vi "Set_Parameter_Instrument (Json).vi"(8 "error in (no error)":errorcluster caption="entrée d'erreur (pas d'erreur)", 10 "Parameter (Json)":string, 11 "Flash_SIN_FP en entrée":refnum<class "Flash_SIN_Test_FW.lvclass">) -> (0 "error out":errorcluster caption="sortie d'erreur", 3 "Flash_SIN_FP en sortie":refnum<class "Flash_SIN_Test_FW.lvclass">)   [LabVIEW 2020, in "Library Test.lvlib" / "Flash_SIN_Test_FW.lvclass"]
uses:
  Flash_SIN_Test_FW.lvclass
  C:/Users/ngarcin/OneDrive - Altyor/Standard TB/Class/Test/Test (Default)/Test (Default).lvclass
  C:/Users/ngarcin/OneDrive - Altyor/Standard TB/Class/Test/Flash_Commander/Flash_Commander.lvclass
  Flash_SIN_Test_FW.lvclass/Flash_SIN_Test_FW.ctl
  JSON API/JSON Value/Set from JSON string.vi
  Flash_Commander/Flash_Commander.lvclass
  JSON API/JSON Value/JSON Value.lvclass
  JSON API/Variant JSON/Variant JSON.lvlib
  JSON API/Get Polymorphic/JSON GetSet.lvlib
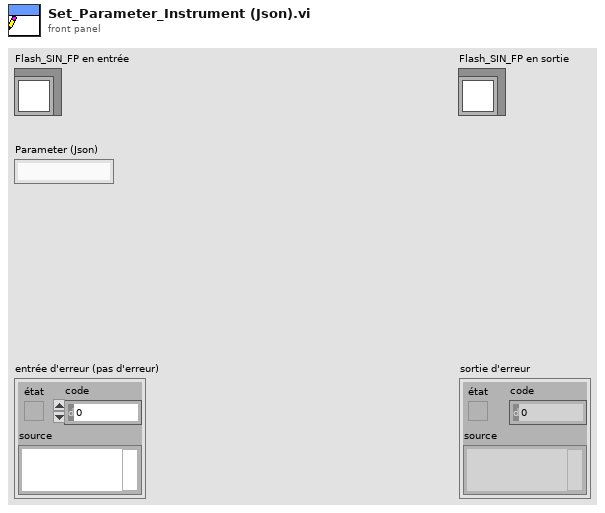
[diagram p1: front panel]
types:
  T1 = cluster{"Firmware path":path, "commander path":path, "Bat path":path}
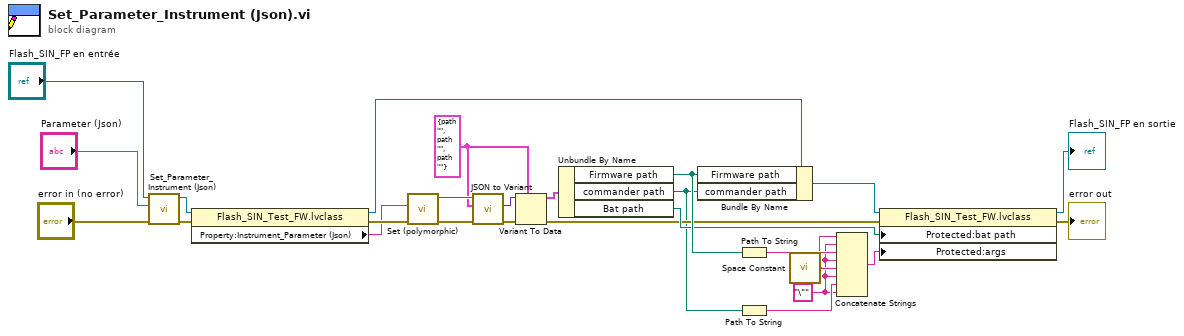
[diagram p0: block diagram]
diagram:
  w1 = "\""
  w13 = T1 {"Firmware path"=path "", "commander path"=path "", "Bat path"=path ""} ("Cluster des données privées de classe")
  n1 = call-parent "Set_Parameter_Instrument (Json).vi"("error in (no error)"="error in (no error)", "Parameter (Json)"="Parameter (Json)", "Test (Default) en entrée"="Flash_SIN_FP en entrée") -> ("error out"=w21:errorcluster, "Test (Default) en sortie"=w20:refnum<class "Flash_SIN_Test_FW.lvclass">)  [unwired: 7 in]
  n2 = property class="Flash_SIN_Test_FW.lvclass"(reference=w20, error in=w21) -> (reference out=w16:refnum<class "Flash_SIN_Test_FW.lvclass">, error out=w19:errorcluster, "Property:Instrument_Parameter (Json)"=w17:string)
  n3 = call-poly "Set (polymorphic).vi"("error in (no error)"=w19, "JSON stream"=w17) -> ("error out"=w24:errorcluster, "JSON Value out"=w26:refnum<class "JSON Value.lvclass">)  [unwired: 7 in, 1 out]
  n4 = call "JSON to Variant.vi"("error in (no error)"=w24, "Variant (Data Type)"=w13, "JSON Value"=w26) -> ("error out"=w25:errorcluster, "Variant out"=w23:variant)  [unwired: 7 in]
  n5 = Variant To Data(error in=w25, type=w13, Variant=w23) -> (data=w15:T1, error out=w3:errorcluster)
  n6 = Unbundle By Name(w15) -> ("Firmware path"=w6:path, "commander path"=w2:path, "Bat path"=w5:path)
  n7 = Bundle By Name(cluster=w16, "Firmware path"=w6, "commander path"=w2) -> (w12:refnum<class "Flash_SIN_Test_FW.lvclass">)
  n8 = Path To String(path=w6) -> (string=w9:string)
  n9 = Path To String(path=w2) -> (string=w7:string)
  n10 = call <vilib>:"Space Constant.vi"() -> ("String"=w8:string)
  n11 = Concatenate Strings(w8, w1, w9, w1, w8, w1, w7, w1) -> (w4:string)
  n12 = property class="Flash_SIN_Test_FW.lvclass"(reference=w12, error in=w3, "Protected:bat path"=w5, "Protected:args"=w4) -> (reference out=→"Flash_SIN_FP en sortie":refnum<class "Flash_SIN_Test_FW.lvclass">, error out=→"error out":errorcluster)
